vi "Recognize Model.vi"(0 "Manufacturer":string, 5 "Model":string, 9 "Model Unwired/Wired":bool, 11 "error in (no error)":errorcluster {"code" format="%.0x"}) -> (6 "Model Out":string, 15 "error out":errorcluster {"code" format="%.0x"})   [LabVIEW 2013]
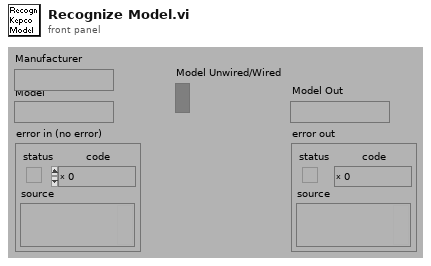
[diagram p1: front panel]
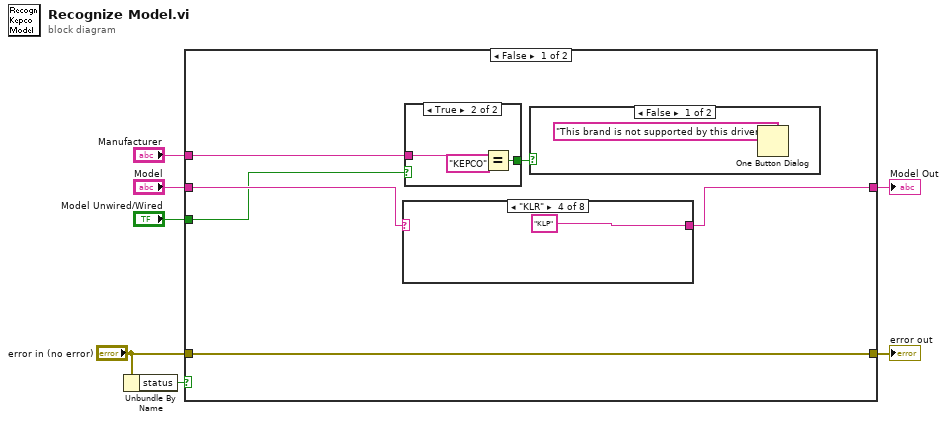
[diagram p0: block diagram]
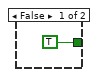
[diagram p2: hidden frame]
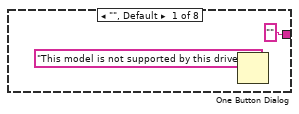
[diagram p3: hidden frame]
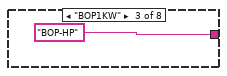
[diagram p5: hidden frame]
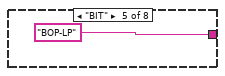
[diagram p6: hidden frame]
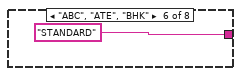
[diagram p7: hidden frame]
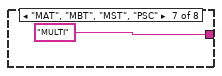
[diagram p8: hidden frame]
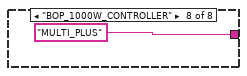
[diagram p9: hidden frame]
diagram:
  n1 = Unbundle By Name("error in (no error)") -> ("status"=w6:bool)
  n2 = case shown="False" w6 {
    tunnel: "error in (no error)" -> [w13 w29]
    tunnel: [w13 w29] -> w5
    tunnel: "Model" -> [w11 w28]
    tunnel: "Manufacturer" -> [w12 _]
    tunnel: [w9 w28] -> w2
    tunnel: "Model Unwired/Wired" -> [w10 _]
    frame False {
      n3 = case shown="\"KLR\"" w11 {
        selector: w11 -> [_ w20 _ _ _ _ _ _]
        tunnel: ["" w20 "BOP-HP" "KLP" "BOP-LP" "STANDARD" "MULTI" "MULTI_PLUS"] -> w9
        frame "", Default {
          n4 = One Button Dialog(message="This model is not supported by this driver!") -> ()  [unwired: 2 out]
        }
        frame "KLP" {
        }
        frame "BOP1KW" {
        }
        frame "KLR" {
        }
        frame "BIT" {
        }
        frame "ABC", "ATE", "BHK" {
        }
        frame "MAT", "MBT", "MST", "PSC" {
        }
        frame "BOP_1000W_CONTROLLER" {
        }
      }
      n5 = case shown="True" w10 {
        tunnel: w12 -> [_ w17]
        tunnel: [TRUE w15] -> w8
        frame False {
        }
        frame True {
          n6 = Equal?(x=w17, y="KEPCO") -> (x = y?=w15:bool)
        }
      }
      n7 = case shown="False" w8 {
        frame False {
          n8 = One Button Dialog(message="This brand is not supported by this driver!") -> ()  [unwired: 2 out]
        }
        frame True {
        }
      }
    }
    frame True {
    }
  }
  "Model Out" <- w2
  "error out" <- w5
